vi "Page_Advanced_Read.vi"(6 "ctlReferences":T1, 8 "error in (no error)":errorcluster, 11 "Class in":refnum<class "IB_MSI.lvclass">) -> (0 "error out":errorcluster, 3 "Class out":refnum<class "IB_MSI.lvclass">)   [LabVIEW 2020, in "IB_MSI.lvclass"]
uses:
  <vilib>/AppBuilder/IB_Classes/MSI/IB_MSI.lvclass
  <vilib>/AppBuilder/IB_Classes/MSI/IB_MSI.lvclass/IB_MSI.ctl
  <vilib>/AppBuilder/IB_Classes/Installer/Installer.lvclass
  <resource>/Framework/Providers/Builds/Installer/Pages/controls/IB_UI_Page_Advanced_References.ctl
  <resource>/Framework/Providers/Builds/Installer/CDK_sTypeDef_SystemRequirements.ctl
  <resource>/Framework/Providers/Common/provcom_BrowseProjectFile2.ctl
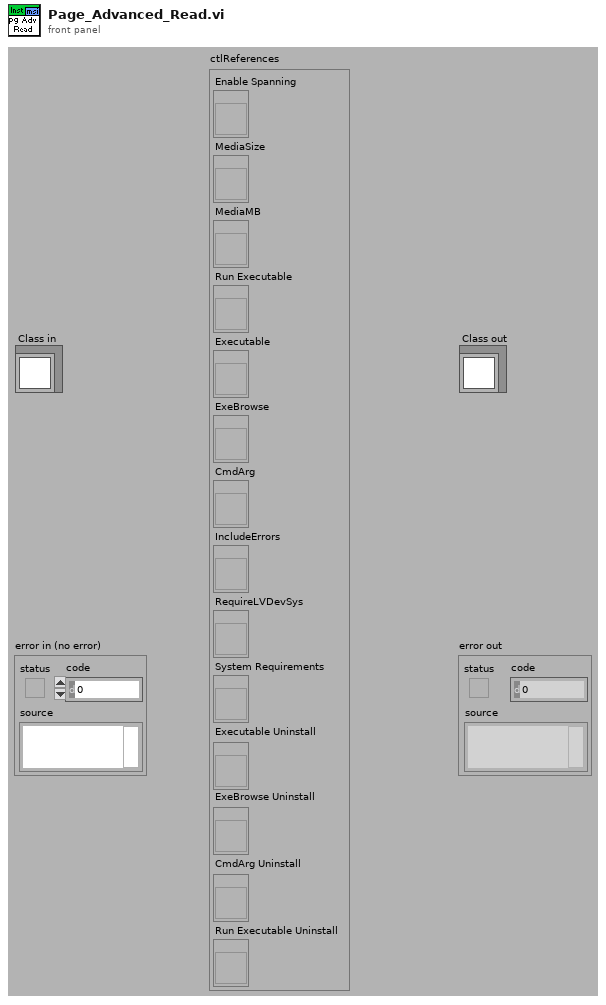
[diagram p1: front panel]
types:
  T1 = typedef "IB_UI_Page_Advanced_References.ctl" = cluster{"Enable Spanning":refnum<vi>, "MediaSize":refnum<vi>, "MediaMB":refnum<vi>, "Run Executable":refnum<vi>, "Executable":refnum<vi>, "ExeBrowse":refnum<vi>, "CmdArg":refnum<vi>, "IncludeErrors":refnum<vi>, "RequireLVDevSys":refnum<vi>, "System Requirements":refnum<vi>, "Executable Uninstall":refnum<vi>, "ExeBrowse Uninstall":refnum<vi>, "CmdArg Uninstall":refnum<vi>, "Run Executable Uninstall":refnum<vi>}
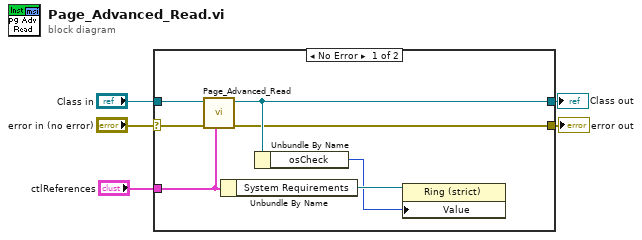
[diagram p0: block diagram]
diagram:
  n1 = case shown="No Error" "error in (no error)" {
    selector: "error in (no error)" -> [w8 w14]
    tunnel: [w7 w14] -> w4
    tunnel: [w9 w13] -> w2
    tunnel: "Class in" -> [w10 w13]
    tunnel: "ctlReferences" -> [w6 _]
    frame No Error {
      n2 = call-parent "Page_Advanced_Read.vi"("ctlReferences"=w6, "error in (no error)"=w8, "Class in"=w10) -> ("error out"=w7:errorcluster, "Class out"=w9:refnum<class "IB_MSI.lvclass">)  [unwired: 7 out]
      n3 = Unbundle By Name(w6) -> ("System Requirements"=w12:refnum<vi>)
      n4 = Unbundle By Name(w9) -> ("osCheck"=w11:i32)
      n5 = property class="Ring (strict)"(reference=w12, "Value"=w11) -> ()  [unwired: 1 in, 2 out]
    }
    frame Error {
    }
  }
  "error out" <- w4
  "Class out" <- w2
